vi "HitrapGUI.setColorStepMotor.vi"(0 "Cluster Refnum":refnum<vi>, 2 "State":T1 caption="index", 5 "error in (no error)":errorcluster) -> (14 "Cluster Refnum Out":refnum<vi>, 19 "error out":errorcluster)   [LabVIEW 2014, in "HitrapGUI.lvlib"]
uses:
  HitrapGUI.lvlib
  CSlibraries/UtilityLib/UtilityLib.valueStatus.ctl
  CSlibraries/UtilityLib/UtilityLib.lvlib
panel:
  in  "?":u8(ring) items=["Undefined", "Open", "Faraday Cup", "MCP"]
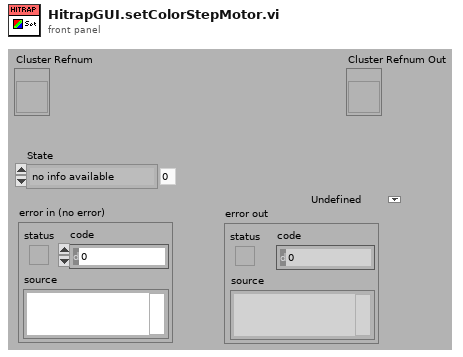
[diagram p1: front panel]
types:
  T1 = typedef "UtilityLib.lvlib/UtilityLib.valueStatus.ctl" = enum16{"no info available", "stand by/off", "on", "warning", "alarm/malfunction", "not implemented", "user action required", "important information", "system default", "control default", "indicator default", "button default"}
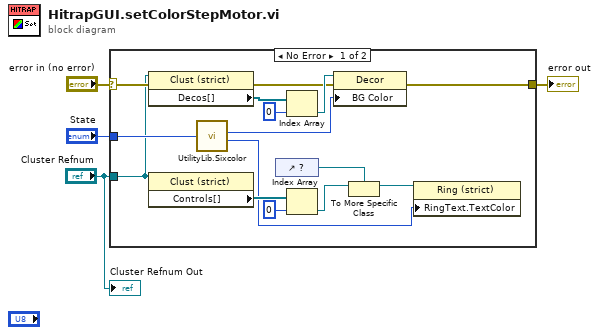
[diagram p0: block diagram]
diagram:
  n1 = case shown="No Error" "error in (no error)" {
    selector: "error in (no error)" -> [w15 w20]
    tunnel: "Cluster Refnum" -> [w6 _]
    tunnel: [w14 w20] -> w3
    tunnel: "State" -> [w12 _]
    frame No Error {
      n2 = property class="Clust (strict)"(reference=w6, error in=w15) -> (error out=w16:errorcluster, "Decos[]"=w19:refnum<vi>[])  [unwired: 1 out]
      n3 = property class="Clust (strict)"(reference=w6) -> ("Controls[]"=w8:refnum<vi>[])  [unwired: 1 in, 2 out]
      n4 = call "UtilityLib.Sixcolor.vi"("State"=w12) -> ("elementBackground"=w13:u32, "elementText"=w5:u32)  [unwired: 2 in, 2 out]
      n5 = control-ref of="?"() -> (w11:refnum<vi>)
      n6 = Index Array(array=w19, index=0) -> (element=w17:refnum<vi>)
      n7 = Index Array(array=w8, index=0) -> (element=w9:refnum<vi>)
      n8 = property class="Decor"(reference=w17, error in=w16, "BG Color"=w13) -> (error out=w14:errorcluster)  [unwired: 1 out]
      n9 = To More Specific Class(target class=w11, reference=w9) -> (specific class reference=w10:refnum<vi>)  [unwired: 1 in, 1 out]
      n10 = property class="Ring (strict)"(reference=w10, "RingText.TextColor"=w5) -> ()  [unwired: 1 in, 2 out]
    }
    frame Error {
    }
  }
  "error out" <- w3
  "Cluster Refnum Out" <- "Cluster Refnum"
